vi "Get Trigger Info.vi"(6 "Device Ref in":T2 format="%.0x", 7 "Trigger Direction":T3, 8 "error in (no error)":errorcluster, 9 "Trigger in":T1 {"Node Data Ref" format="%.0x"; "Node ID" format="%.0x"}, 10 "Channel Refs in":T4 {"Trigger Data Refs"."Data Reference" format="%.0x"; "Trigger Chan Refs" format="%.0x"; "System Time"."Get Date-Time Channel Data Ref" format="%.0x"; "System Time"."Absolute Time Channel Data Ref" format="%.0x"; "System Time"."Channel Data Reference" format="%.0x"; "Status Data Refs"."Data Reference" format="%.0x"; "Command Data Refs"."Data Reference" format="%.0x"; "Status Chan Refs" format="%.0x"; "Command Chan Refs" format="%.0x"}, 11 "Item Ref in":T2 format="%.0x") -> (0 "error out":errorcluster, 1 "Trigger out":T1 {"Node Data Ref" format="%.0x"; "Node ID" format="%.0x"}, 2 "Channel Refs out":T4 {"Trigger Data Refs"."Data Reference" format="%.0x"; "Trigger Chan Refs" format="%.0x"; "System Time"."Get Date-Time Channel Data Ref" format="%.0x"; "System Time"."Absolute Time Channel Data Ref" format="%.0x"; "System Time"."Channel Data Reference" format="%.0x"; "Status Data Refs"."Data Reference" format="%.0x"; "Command Data Refs"."Data Reference" format="%.0x"; "Status Chan Refs" format="%.0x"; "Command Chan Refs" format="%.0x"}, 3 "Item Ref out":T2 format="%.0x", 5 "Multi-trig":bool)   [LabVIEW 2012, in "Waveform Data Logger Engine.lvlib"]
uses:
  Waveform Data Logger Engine.lvlib
  Types/Channels.ctl
  <vilib>/NI Veristand/Custom Device API/Custom Device Item Ref.ctl
  <vilib>/NI Veristand/Custom Device API/Block Data Reference.ctl
  <vilib>/NI Veristand/Custom Device API/Data Reference.ctl
  Types/System Time.ctl
  Shared/Types/Trigger Direction.ctl
  Types/Trigger Settings.ctl
  Classes/Triggers/Trigger/Trigger.lvclass
  Shared/Types/Start Trigger.ctl
  Classes/Triggers/Boolean Evaluation Trigger/Operand.ctl
  Shared/Types/Stop Trigger.ctl
  <vilib>/NI Veristand/Custom Device API/Data Access Type.ctl
  Shared/Globals/Property Strings.vi
  <vilib>/NI Veristand/Custom Device API/Get Item Property (U16).vi
  <vilib>/NI Veristand/Custom Device API/Get Item Property (Boolean).vi
  <vilib>/NI Veristand/Custom Device API/Get Item Property (Double).vi
  <vilib>/NI Veristand/Custom Device API/Get Item Property (Dependent Node Pointer).vi
  <vilib>/NI VeriStand/Custom Device API/Custom Device API.lvlib
  Shared/Waveform Data Logger Shared.lvlib
  Classes/Triggers/Default Trigger/Default Trigger.lvclass
  Classes/Triggers/Digital Edge Trigger/Digital Edge Trigger.lvclass
  Classes/Triggers/Analog Edge Trigger/Analog Edge Trigger.lvclass
  Classes/Triggers/In Range Trigger/In Range Trigger.lvclass
  Classes/Triggers/Value Change Trigger/Value Change Trigger.lvclass
  Classes/Triggers/Boolean Evaluation Trigger/Boolean Evaluation Trigger.lvclass
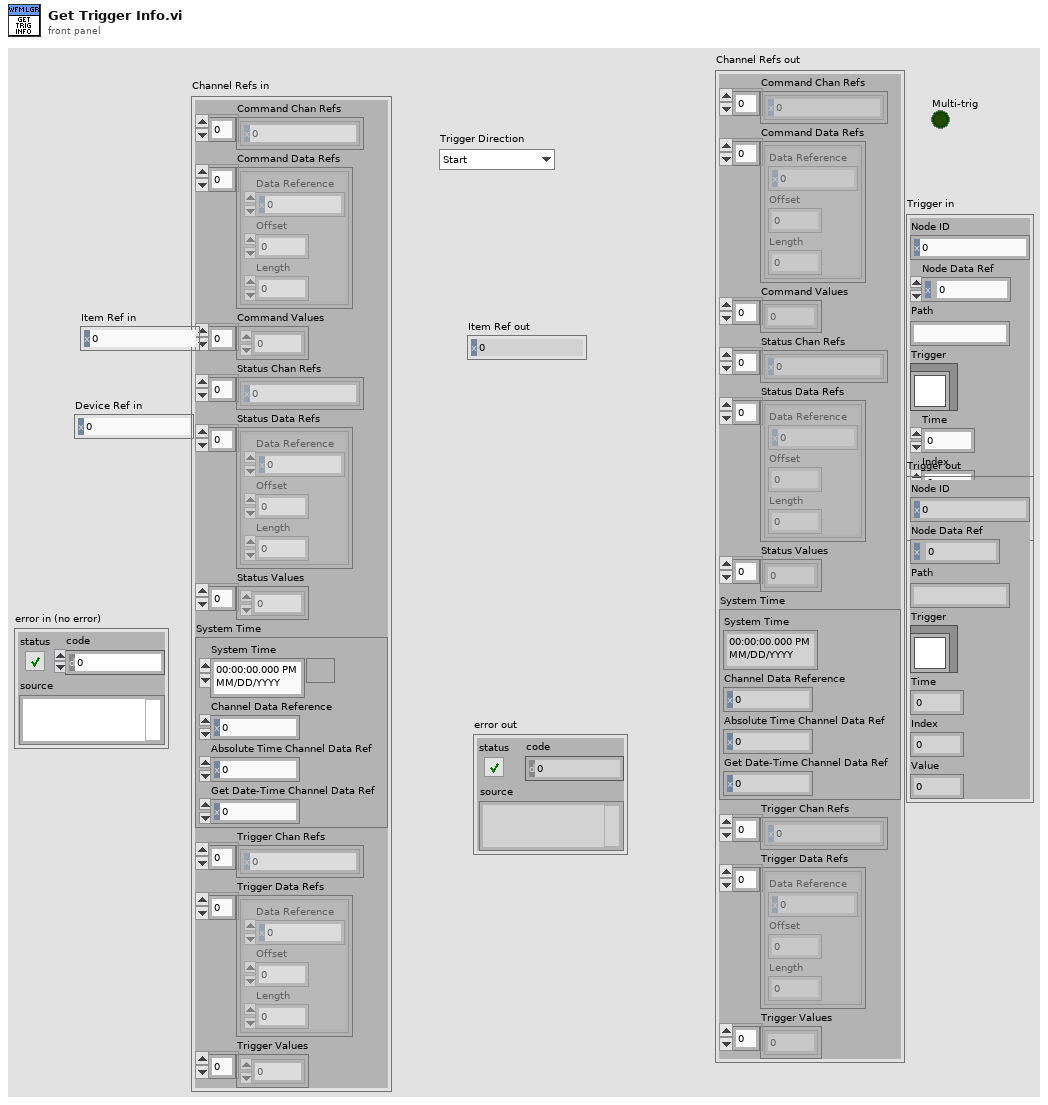
[diagram p1: front panel]
types:
  T1 = typedef "Waveform Data Logger Engine.lvlib/Trigger Settings.ctl" = cluster{"Node ID":T2, "Node Data Ref":i32, "Path":string, "Trigger":refnum<class "Trigger.lvclass">, "Time":dbl, "Index":i32, "Value":dbl}
  T2 = typedef "Custom Device API.lvlib/Custom Device Item Ref.ctl" = u64
  T3 = typedef "Waveform Data Logger Shared.lvlib/Trigger Direction.ctl" = enum16{"Start", "Stop"}
  T4 = typedef "Waveform Data Logger Engine.lvlib/Channels.ctl" = cluster{"Command Chan Refs":T2[], "Command Data Refs":T5[], "Command Values":dbl[], "Status Chan Refs":T2[], "Status Data Refs":T5[], "Status Values":dbl[], "System Time":T7, "Trigger Chan Refs":T2[], "Trigger Data Refs":T5[], "Trigger Values":dbl[]}
  T5 = typedef "Custom Device API.lvlib/Block Data Reference.ctl" = cluster{"Data Reference":T6, "Offset":i32, "Length":i32}
  T6 = typedef "Custom Device API.lvlib/Data Reference.ctl" = i32
  T7 = typedef "Waveform Data Logger Engine.lvlib/System Time.ctl" = cluster{"System Time":timestamp, "Data Reference":T6, "Absolute Time Channel Data Ref":T6, "Get Date-Time Channel Data Ref":T6}
  T8 = typedef "Custom Device API.lvlib/Data Access Type.ctl" = enum16{"Read", "Write"}
  T9 = typedef "Waveform Data Logger Shared.lvlib/Start Trigger.ctl" = enum16{"Start immediately", "Start on digital edge", "Start on analog edge", "Start when in range", "Start when out of range", "Start on value change", "Start when Boolean condition is true"}
  T10 = typedef "Waveform Data Logger Engine.lvlib/Boolean Evaluation Trigger.lvclass/Operand.ctl" = enum16{"==", "!=", "<", "<=", ">", ">="}
  T11 = typedef "Waveform Data Logger Shared.lvlib/Stop Trigger.ctl" = enum16{"Log indefinitely", "Stop after duration", "Stop on digital edge", "Stop on analog edge", "Stop when in range", "Stop when out of range", "Stop on value change", "Stop when Boolean condition is true"}
  T12 = typedef "Waveform Data Logger Shared.lvlib/Default Trigger.ctl" = cluster{"Default State":bool}
  T13 = typedef "Waveform Data Logger Shared.lvlib/Digital Trigger.ctl" = cluster{"Edge":enum16{"Rising", "Falling"}}
  T14 = typedef "Waveform Data Logger Shared.lvlib/Analog Trigger.ctl" = cluster{"Strict edge":bool, "Slope":enum16{"Rising", "Falling"}, "Threshold":dbl}
  T15 = typedef "Waveform Data Logger Shared.lvlib/In Range Trigger.ctl" = cluster{"High limit":dbl, "Low limit":dbl, "Invert?":bool}
  T16 = typedef "Waveform Data Logger Shared.lvlib/Value Change Trigger.ctl" = cluster{"Deadband":dbl}
  T17 = typedef "Waveform Data Logger Shared.lvlib/Boolean Trigger.ctl" = cluster{"Value":dbl, "Operand":enum16{"Equal to", "Not equal to", "Less than", "Less than or equal", "Greater than", "Greater than or equal"}}
  T18 = enum16{"Equal to", "Not equal to", "Less than", "Less than or equal", "Greater than", "Greater than or equal"}
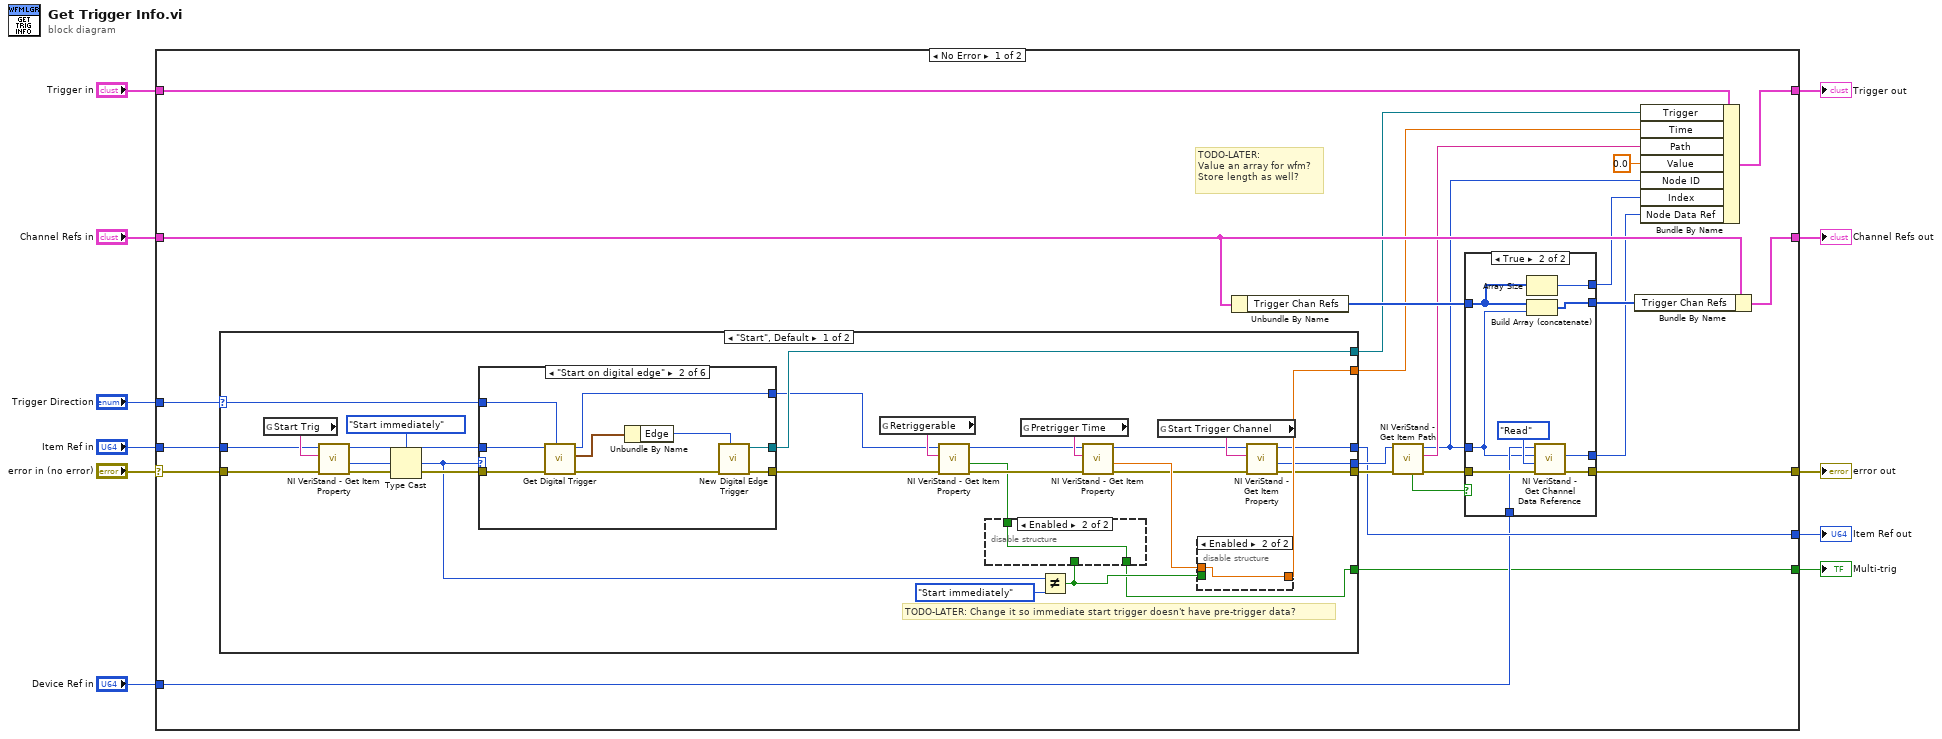
[diagram p0: block diagram]
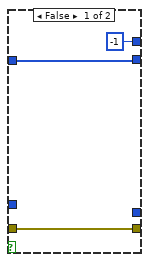
[diagram p2: hidden frame]
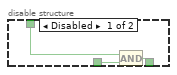
[diagram p3: hidden frame]
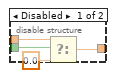
[diagram p4: hidden frame]
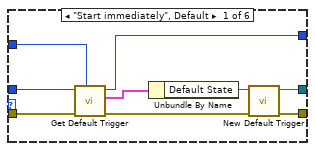
[diagram p5: hidden frame]
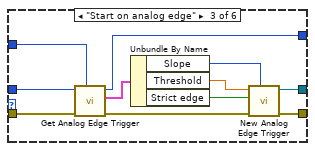
[diagram p6: hidden frame]
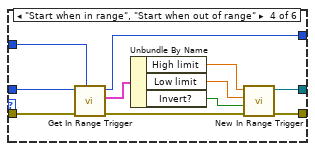
[diagram p7: hidden frame]
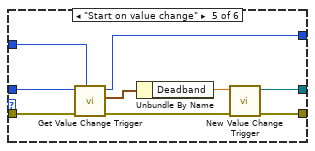
[diagram p8: hidden frame]
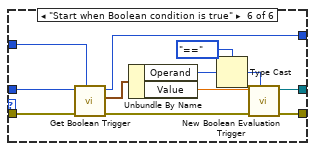
[diagram p9: hidden frame]
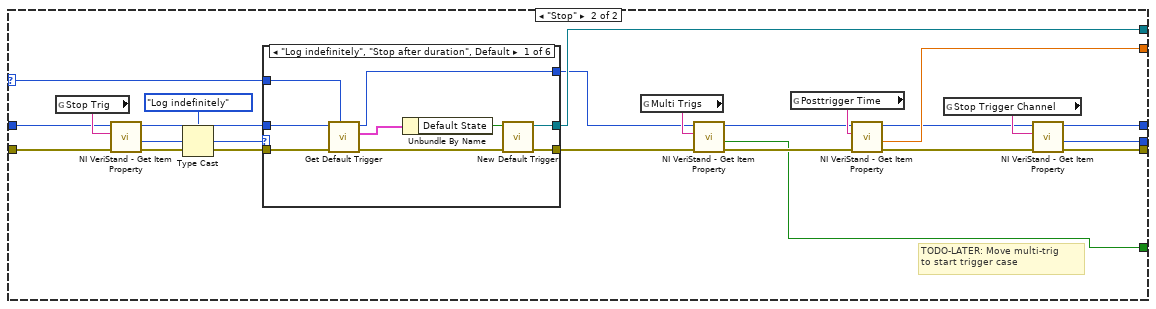
[diagram p10: hidden frame]
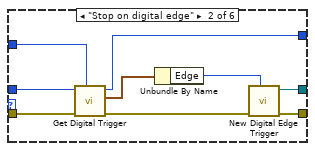
[diagram p11: hidden frame]
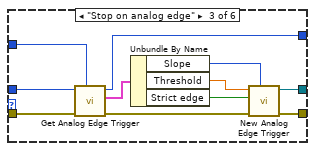
[diagram p12: hidden frame]
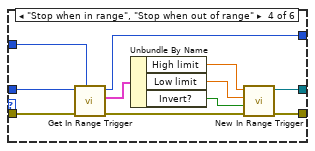
[diagram p13: hidden frame]
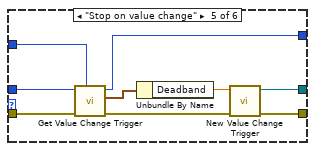
[diagram p14: hidden frame]
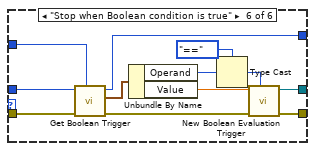
[diagram p15: hidden frame]
diagram:
  n1 = case shown="No Error" "error in (no error)" {
    selector: "error in (no error)" -> [w33 w234]
    tunnel: "Channel Refs in" -> [w32 w232]
    tunnel: [w20 w234] -> w9
    tunnel: "Device Ref in" -> [w18 _]
    tunnel: "Trigger Direction" -> [w35 _]
    tunnel: "Item Ref in" -> [w34 w233]
    tunnel: "Trigger in" -> [w29 w231]
    tunnel: [w22 w232] -> w4
    tunnel: [w19 w233] -> w3
    tunnel: [w17 w231] -> w2
    tunnel: [w12 _] -> w1
    frame No Error {
      # "TODO-LATER:\nValue an array for wfm?\nStore length as well?"
      n2 = case shown="\"Start\", Default" w35 {
        selector: w35 -> [w69 w161]
        tunnel: w34 -> [w68 w163]
        tunnel: w33 -> [w67 w164]
        tunnel: [w60 w160] -> w28
        tunnel: [w65 w159] -> w27
        tunnel: [w61 w155] -> w30
        tunnel: [w59 w154] -> w25
        tunnel: [w58 w153] -> w19
        tunnel: [w48 w146] -> w12
        frame "Start", Default {
          # "TODO-LATER: Change it so immediate start trigger doesn't have pre-trigger data?"
          n3 = global read "Property Strings.vi" "Start Trig"() -> (w75:string)
          n4 = call-poly <vilib>:"NI VeriStand - Get Item Property.vi"("error in (no error)"=w67, "Property Name"=w75, "Item Ref in"=w68) -> ("error out"=w72:errorcluster, "Value"=w74:u16, "Item Ref out"=w71:T2)  [unwired: 1 in, 5 out]
          n5 = Type Cast(type=Start_Trigger."Start immediately" ("Value (Signaling)"), x=w74) -> (*(type *) &x=w57:T9)
          n6 = case shown="\"Start on digital edge\"" w57 {
            tunnel: w72 -> [w93 w101 w112 w123 w133 w145]
            tunnel: w71 -> [w92 w102 w113 w124 w125 w144]
            tunnel: [w88 w95 w104 w115 w127 w135] -> w54
            tunnel: [w87 w97 w105 w116 w128 w136] -> w55
            tunnel: [w86 w96 w106 w117 w129 w137] -> w60
            tunnel: w69 -> [w85 w94 w103 w114 w126 w134]
            frame "Start immediately", Default {
              n7 = call "Get Default Trigger.vi"("Trigger Direction"=w85, "error in (no error)"=w93, "Item Ref in"=w92) -> ("error out"=w90:errorcluster, "Default Trigger"=w91:T12, "Item Ref out"=w88:T2)  [unwired: 6 in]
              n8 = Unbundle By Name(w91) -> ("Default State"=w89:bool)
              n9 = call "New Default Trigger.vi"("error in (no error)"=w90, "Default State"=w89) -> ("error out"=w87:errorcluster, "Default Trigger out"=w86:refnum<class "Default Trigger.lvclass">)  [unwired: 8 in]
            }
            frame "Start on digital edge" {
              n10 = call "Get Digital Trigger.vi"("Trigger Direction"=w94, "error in (no error)"=w101, "Item Ref in"=w102) -> ("error out"=w98:errorcluster, "Digital Trigger"=w100:T13, "Item Ref out"=w95:T2)  [unwired: 6 in]
              n11 = Unbundle By Name(w100) -> ("Edge"=w99:enum16{"Rising", "Falling"})
              n12 = call "New Digital Edge Trigger.vi"("Slope"=w99, "error in (no error)"=w98) -> ("error out"=w97:errorcluster, "Digital Edge Trigger out"=w96:refnum<class "Digital Edge Trigger.lvclass">)  [unwired: 8 in]
            }
            frame "Start on analog edge" {
              n13 = call "Get Analog Edge Trigger.vi"("Trigger Direction"=w103, "error in (no error)"=w112, "Item Ref in"=w113) -> ("error out"=w111:errorcluster, "Analog Trigger"=w110:T14, "Item Ref out"=w104:T2)  [unwired: 6 in]
              n14 = Unbundle By Name(w110) -> ("Slope"=w109:enum16{"Rising", "Falling"}, "Threshold"=w107:dbl, "Strict edge"=w108:bool)
              n15 = call "New Analog Edge Trigger.vi"("Slope"=w109, "error in (no error)"=w111, "Strict Edge"=w108, "Threshold"=w107) -> ("error out"=w105:errorcluster, "Analog Edge Trigger out"=w106:refnum<class "Analog Edge Trigger.lvclass">)  [unwired: 6 in]
            }
            frame "Start when in range", "Start when out of range" {
              n16 = call "Get In Range Trigger.vi"("Trigger Direction"=w114, "error in (no error)"=w123, "Item Ref in"=w124) -> ("error out"=w120:errorcluster, "In Range Trigger"=w122:T15, "Item Ref out"=w115:T2)  [unwired: 6 in]
              n17 = Unbundle By Name(w122) -> ("High limit"=w121:dbl, "Low limit"=w118:dbl, "Invert?"=w119:bool)
              n18 = call "New In Range Trigger.vi"("error in (no error)"=w120, "Invert"=w119, "Lower Limit"=w118, "Upper Limit"=w121) -> ("error out"=w116:errorcluster, "In Range Trigger out"=w117:refnum<class "In Range Trigger.lvclass">)  [unwired: 6 in]
            }
            frame "Start on value change" {
              n19 = call "Get Value Change Trigger.vi"("Trigger Direction"=w126, "error in (no error)"=w133, "Item Ref in"=w125) -> ("error out"=w132:errorcluster, "Value Change Trigger"=w131:T16, "Item Ref out"=w127:T2)  [unwired: 6 in]
              n20 = Unbundle By Name(w131) -> ("Deadband"=w130:dbl)
              n21 = call "New Value Change Trigger.vi"("error in (no error)"=w132, "Deadband"=w130) -> ("error out"=w128:errorcluster, "Value Change Trigger out"=w129:refnum<class "Value Change Trigger.lvclass">)  [unwired: 8 in]
            }
            frame "Start when Boolean condition is true" {
              n22 = call "Get Boolean Trigger.vi"("Trigger Direction"=w134, "error in (no error)"=w145, "Item Ref in"=w144) -> ("error out"=w143:errorcluster, "Boolean Trigger"=w142:T17, "Item Ref out"=w135:T2)  [unwired: 6 in]
              n23 = Unbundle By Name(w142) -> ("Operand"=w141:T18, "Value"=w138:dbl)
              n24 = Type Cast(type=Operand."==" ("Operand"), x=w141) -> (*(type *) &x=w139:T10)
              n25 = call "New Boolean Evaluation Trigger.vi"("Operand"=w139, "error in (no error)"=w143, "Value"=w138) -> ("error out"=w136:errorcluster, "Boolean Evaluation Trigger out"=w137:refnum<class "Boolean Evaluation Trigger.lvclass">)  [unwired: 7 in]
            }
          }
          n26 = global read "Property Strings.vi" "Retriggerable"() -> (w56:string)
          n27 = call-poly <vilib>:"NI VeriStand - Get Item Property.vi"("error in (no error)"=w55, "Property Name"=w56, "Item Ref in"=w54) -> ("error out"=w53:errorcluster, "Value"=w49:bool, "Item Ref out"=w52:T2)  [unwired: 1 in, 5 out]
          n28 = global read "Property Strings.vi" "Pretrigger Time"() -> (w70:string)
          n29 = Not Equal?(x=w57, y=Start_Trigger."Start immediately" ("Value (Signaling)")) -> (x != y?=w50:bool)
          n30 = disable-structure shown="Enabled" {
            disable-tunnel: w50 -> [w78 _]
            disable-tunnel: w49 -> [w77 w79]
            disable-tunnel: [w76 w79] -> w48
            frame Disabled {
              n31 = And(x=w77, y=w78) -> (x .and. y?=w76:bool)
            }
            frame Enabled {
            }
          }
          n32 = call-poly <vilib>:"NI VeriStand - Get Item Property.vi"("error in (no error)"=w53, "Property Name"=w70, "Item Ref in"=w52) -> ("error out"=w63:errorcluster, "Value"=w66:dbl, "Item Ref out"=w62:T2)  [unwired: 1 in, 5 out]
          n33 = global read "Property Strings.vi" "Start Trigger Channel"() -> (w64:string)
          n34 = disable-structure shown="Enabled" {
            disable-tunnel: w66 -> [w83 w84]
            disable-tunnel: [w82 w84] -> w65
            disable-tunnel: w50 -> [w80 _]
            frame Disabled {
              n35 = Select(t=w83, s=w80, f=0.0) -> (s? t:f=w82:dbl)
            }
            frame Enabled {
            }
          }
          n36 = call-poly <vilib>:"NI VeriStand - Get Item Property.vi"("error in (no error)"=w63, "Property Name"=w64, "Item Ref in"=w62) -> ("error out"=w61:errorcluster, "Dependent Node Ref"=w59:T2, "Item Ref out"=w58:T2)  [unwired: 6 out]
        }
        frame "Stop" {
          # "TODO-LATER: Move multi-trig\nto start trigger case"
          n37 = global read "Property Strings.vi" "Stop Trig"() -> (w166:string)
          n38 = call-poly <vilib>:"NI VeriStand - Get Item Property.vi"("error in (no error)"=w164, "Property Name"=w166, "Item Ref in"=w163) -> ("error out"=w168:errorcluster, "Value"=w167:u16, "Item Ref out"=w169:T2)  [unwired: 1 in, 5 out]
          n39 = Type Cast(type=Stop_Trigger."Log indefinitely" ("Stop Trigger"), x=w167) -> (*(type *) &x=w152:T11)
          n40 = case shown="\"Log indefinitely\", \"Stop after duration\", Default" w152 {
            tunnel: w168 -> [w178 w186 w197 w208 w217 w230]
            tunnel: w169 -> [w177 w187 w198 w209 w218 w229]
            tunnel: [w173 w180 w189 w200 w211 w220] -> w150
            tunnel: [w172 w182 w190 w201 w212 w221] -> w149
            tunnel: [w171 w181 w191 w202 w213 w222] -> w160
            tunnel: w161 -> [w170 w179 w188 w199 w210 w219]
            frame "Log indefinitely", "Stop after duration", Default {
              n41 = call "Get Default Trigger.vi"("Trigger Direction"=w170, "error in (no error)"=w178, "Item Ref in"=w177) -> ("error out"=w175:errorcluster, "Default Trigger"=w176:T12, "Item Ref out"=w173:T2)  [unwired: 6 in]
              n42 = Unbundle By Name(w176) -> ("Default State"=w174:bool)
              n43 = call "New Default Trigger.vi"("error in (no error)"=w175, "Default State"=w174) -> ("error out"=w172:errorcluster, "Default Trigger out"=w171:refnum<class "Default Trigger.lvclass">)  [unwired: 8 in]
            }
            frame "Stop on digital edge" {
              n44 = call "Get Digital Trigger.vi"("Trigger Direction"=w179, "error in (no error)"=w186, "Item Ref in"=w187) -> ("error out"=w183:errorcluster, "Digital Trigger"=w185:T13, "Item Ref out"=w180:T2)  [unwired: 6 in]
              n45 = Unbundle By Name(w185) -> ("Edge"=w184:enum16{"Rising", "Falling"})
              n46 = call "New Digital Edge Trigger.vi"("Slope"=w184, "error in (no error)"=w183) -> ("error out"=w182:errorcluster, "Digital Edge Trigger out"=w181:refnum<class "Digital Edge Trigger.lvclass">)  [unwired: 8 in]
            }
            frame "Stop on analog edge" {
              n47 = call "Get Analog Edge Trigger.vi"("Trigger Direction"=w188, "error in (no error)"=w197, "Item Ref in"=w198) -> ("error out"=w196:errorcluster, "Analog Trigger"=w195:T14, "Item Ref out"=w189:T2)  [unwired: 6 in]
              n48 = Unbundle By Name(w195) -> ("Slope"=w194:enum16{"Rising", "Falling"}, "Threshold"=w192:dbl, "Strict edge"=w193:bool)
              n49 = call "New Analog Edge Trigger.vi"("Slope"=w194, "error in (no error)"=w196, "Strict Edge"=w193, "Threshold"=w192) -> ("error out"=w190:errorcluster, "Analog Edge Trigger out"=w191:refnum<class "Analog Edge Trigger.lvclass">)  [unwired: 6 in]
            }
            frame "Stop when in range", "Stop when out of range" {
              n50 = call "Get In Range Trigger.vi"("Trigger Direction"=w199, "error in (no error)"=w208, "Item Ref in"=w209) -> ("error out"=w205:errorcluster, "In Range Trigger"=w207:T15, "Item Ref out"=w200:T2)  [unwired: 6 in]
              n51 = Unbundle By Name(w207) -> ("High limit"=w206:dbl, "Low limit"=w203:dbl, "Invert?"=w204:bool)
              n52 = call "New In Range Trigger.vi"("error in (no error)"=w205, "Invert"=w204, "Lower Limit"=w203, "Upper Limit"=w206) -> ("error out"=w201:errorcluster, "In Range Trigger out"=w202:refnum<class "In Range Trigger.lvclass">)  [unwired: 6 in]
            }
            frame "Stop on value change" {
              n53 = call "Get Value Change Trigger.vi"("Trigger Direction"=w210, "error in (no error)"=w217, "Item Ref in"=w218) -> ("error out"=w216:errorcluster, "Value Change Trigger"=w215:T16, "Item Ref out"=w211:T2)  [unwired: 6 in]
              n54 = Unbundle By Name(w215) -> ("Deadband"=w214:dbl)
              n55 = call "New Value Change Trigger.vi"("error in (no error)"=w216, "Deadband"=w214) -> ("error out"=w212:errorcluster, "Value Change Trigger out"=w213:refnum<class "Value Change Trigger.lvclass">)  [unwired: 8 in]
            }
            frame "Stop when Boolean condition is true" {
              n56 = call "Get Boolean Trigger.vi"("Trigger Direction"=w219, "error in (no error)"=w230, "Item Ref in"=w229) -> ("error out"=w228:errorcluster, "Boolean Trigger"=w227:T17, "Item Ref out"=w220:T2)  [unwired: 6 in]
              n57 = Unbundle By Name(w227) -> ("Operand"=w226:T18, "Value"=w223:dbl)
              n58 = Type Cast(type=Operand."==" ("Operand"), x=w226) -> (*(type *) &x=w224:T10)
              n59 = call "New Boolean Evaluation Trigger.vi"("Operand"=w224, "error in (no error)"=w228, "Value"=w223) -> ("error out"=w221:errorcluster, "Boolean Evaluation Trigger out"=w222:refnum<class "Boolean Evaluation Trigger.lvclass">)  [unwired: 7 in]
            }
          }
          n60 = global read "Property Strings.vi" "Multi Trigs"() -> (w151:string)
          n61 = call-poly <vilib>:"NI VeriStand - Get Item Property.vi"("error in (no error)"=w149, "Property Name"=w151, "Item Ref in"=w150) -> ("error out"=w147:errorcluster, "Value"=w146:bool, "Item Ref out"=w148:T2)  [unwired: 1 in, 5 out]
          n62 = global read "Property Strings.vi" "Posttrigger Time"() -> (w162:string)
          n63 = call-poly <vilib>:"NI VeriStand - Get Item Property.vi"("error in (no error)"=w147, "Property Name"=w162, "Item Ref in"=w148) -> ("error out"=w156:errorcluster, "Value"=w159:dbl, "Item Ref out"=w157:T2)  [unwired: 1 in, 5 out]
          n64 = global read "Property Strings.vi" "Stop Trigger Channel"() -> (w158:string)
          n65 = call-poly <vilib>:"NI VeriStand - Get Item Property.vi"("error in (no error)"=w156, "Property Name"=w158, "Item Ref in"=w157) -> ("error out"=w155:errorcluster, "Dependent Node Ref"=w154:T2, "Item Ref out"=w153:T2)  [unwired: 6 out]
        }
      }
      n66 = Unbundle By Name(w32) -> ("Trigger Chan Refs"=w31:T2[])
      n67 = call <vilib>:"NI VeriStand - Get Item Path.vi"("error in (no error)"=w30, "Item Ref in"=w25) -> ("error out"=w24:errorcluster, "Path"=w26:string, "Item Ref out"=w16:T2, "Found"=w14:bool)  [unwired: 6 in]
      n68 = case shown="True" w14 {
        tunnel: w31 -> [w38 w40]
        tunnel: w24 -> [w37 w46]
        tunnel: [w38 w45] -> w23
        tunnel: [w37 w44] -> w20
        tunnel: w18 -> [_ w43]
        tunnel: w16 -> [_ w42]
        tunnel: [_ w41] -> w15
        tunnel: [-1 w39] -> w13
        frame False {
        }
        frame True {
          n69 = Array Size(array=w40) -> (size(s)=w39:i32)
          n70 = Build Array (concatenate)(w40, w42) -> (w45:T2[])
          n71 = call <vilib>:"NI VeriStand - Get Channel Data Reference.vi"("error in (no error)"=w46, "Access"=Data_Access_Type."Read", "Channel Ref in"=w42, "Device Ref in"=w43) -> ("error out"=w44:errorcluster, "Channel Data Reference"=w41:T6)  [unwired: 5 in, 1 out]
        }
      }
      n72 = Bundle By Name(cluster=w32, "Trigger Chan Refs"=w23) -> (w22:T4)
      n73 = Bundle By Name(cluster=w29, "Trigger"=w28, "Time"=w27, "Path"=w26, "Value"=0.0, "Node ID"=w16, "Index"=w13, "Node Data Ref"=w15) -> (w17:T1)
    }
    frame Error {
    }
  }
  "error out" <- w9
  "Channel Refs out" <- w4
  "Item Ref out" <- w3
  "Trigger out" <- w2
  "Multi-trig" <- w1
